vi "main_serial_communication_2.vi"() -> ()   [LabVIEW 2015]
panel:
  in  "?":bool
  out "flow 3":sgl
  out "flow 2":sgl
  out "flow":sgl
  in  "delay (ms)":u32=500
  in  "MFC 3":bool
  in  "MFC 2":bool
  in  "MFC 1":bool
  out "Center 2":sgl(graph)
  out "호퍼2":sgl(graph)
  out "호퍼1":sgl(graph)
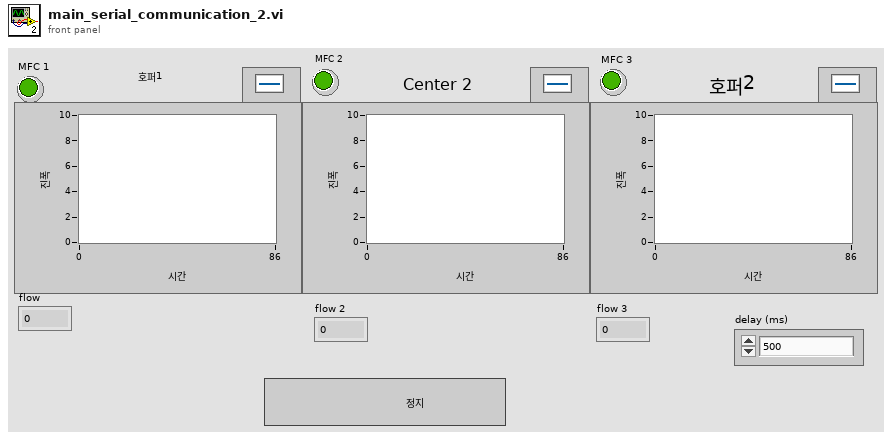
[diagram p1: front panel]
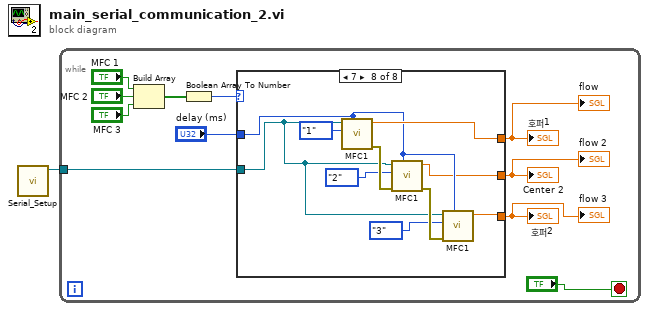
[diagram p0: block diagram]
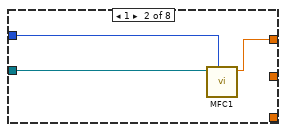
[diagram p3: hidden frame]
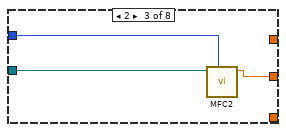
[diagram p4: hidden frame]
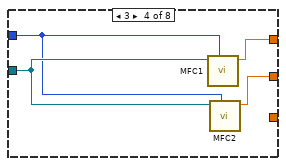
[diagram p5: hidden frame]
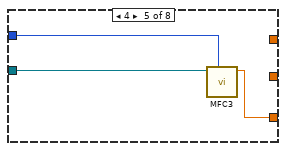
[diagram p6: hidden frame]
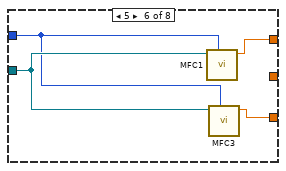
[diagram p7: hidden frame]
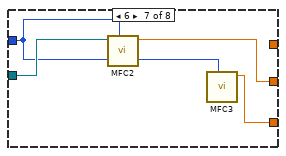
[diagram p8: hidden frame]
diagram:
  n1 = call "Serial_Setup.vi"() -> ("VISA resource name out"=w1:refnum<visa-resource-name>)  [unwired: 10 in, 1 out]
  n2 = while {
    tunnel: w1 -> [w4]
    stop <- "?" stop-if-true
    n3 = Build Array("MFC 1", "MFC 2", "MFC 3") -> (w10:bool[])
    n4 = Boolean Array To Number(Boolean array=w10) -> (number=w8:u32)
    n5 = case shown="7" w8 {
      tunnel: [_ w14 _ w21 _ w27 _ w43] -> w7
      tunnel: [_ _ _ _ w23 w26 w30 w35] -> w5
      tunnel: [_ _ w18 w20 _ _ w31 w34] -> w6
      tunnel: w4 -> [_ w15 w17 w22 w25 w29 w33 w37]
      tunnel: "delay (ms)" -> [_ w13 w16 w19 w24 w28 w32 w36]
      frame 0, Default {
      }
      frame 1 {
        n6 = call "MFC1.vi"("delay (ms)"=w13, "Port"=w15) -> ("flow"=w14:sgl)  [unwired: 8 in, 1 out]
      }
      frame 2 {
        n7 = call "MFC2.vi"("delay (ms)"=w16, "Port"=w17) -> ("flow"=w18:sgl)  [unwired: 9 in]
      }
      frame 3 {
        n8 = call "MFC1.vi"("delay (ms)"=w19, "Port"=w22) -> ("flow"=w21:sgl)  [unwired: 8 in, 1 out]
        n9 = call "MFC2.vi"("delay (ms)"=w19, "Port"=w22) -> ("flow"=w20:sgl)  [unwired: 9 in]
      }
      frame 4 {
        n10 = call "MFC3.vi"("delay (ms)"=w24, "Port"=w25) -> ("flow"=w23:sgl)  [unwired: 9 in]
      }
      frame 5 {
        n11 = call "MFC1.vi"("delay (ms)"=w28, "Port"=w29) -> ("flow"=w27:sgl)  [unwired: 8 in, 1 out]
        n12 = call "MFC3.vi"("delay (ms)"=w28, "Port"=w29) -> ("flow"=w26:sgl)  [unwired: 9 in]
      }
      frame 6 {
        n13 = call "MFC2.vi"("delay (ms)"=w32, "Port"=w33) -> ("flow"=w31:sgl)  [unwired: 9 in]
        n14 = call "MFC3.vi"("delay (ms)"=w32) -> ("flow"=w30:sgl)  [unwired: 10 in]
      }
      frame 7 {
        n15 = call "MFC1.vi"("delay (ms)"=w36, "열거형"=enum16{"1", "2", "3"}."1", "Port"=w37) -> ("error out"=w42:errorcluster, "flow"=w43:sgl)  [unwired: 7 in]
        n16 = call "MFC1.vi"("delay (ms)"=w36, "error in (no error)"=w42, "열거형"=enum16{"1", "2", "3"}."2", "Port"=w37) -> ("error out"=w41:errorcluster, "flow"=w34:sgl)  [unwired: 6 in]
        n17 = call "MFC1.vi"("delay (ms)"=w36, "error in (no error)"=w41, "열거형"=enum16{"1", "2", "3"}."3", "Port"=w37) -> ("flow"=w35:sgl)  [unwired: 6 in, 1 out]
      }
    }
    "호퍼1" <- w7
    "호퍼2" <- w5
    "Center 2" <- w6
    "flow" <- w7
    "flow 2" <- w6
    "flow 3" <- w5
  }
